vi "ThermoV_ControlSweep_2VO_160717.vi"() -> ()   [LabVIEW 2013]
uses:
  <vilib>/Analysis/baseanly.llb/Mean (DBL).vi
  <vilib>/Analysis/NI_AALBase.lvlib
panel:
  out "time/(60*13) indicator":dbl
  out "VGate Mod10 indicator":dbl
  in  "Operate HVpp\nOutput Timer":bool caption="Reset"
  out "modular 13":dbl
  in  "Number of seconds for \neach HVpp case state":dbl=30.0
  out "Elapsed Time (s)":dbl
  out "DC Value":dbl[](array[numeric]) format="%#.6f"
  in  "How many samples\nto average?":dbl
  in  "Saving Avg?":bool
  in  "Filename":path=path "trial_1.lvm"
  out "Samples Indicator":dbl
  in  "STOP":bool
  in  "Save Waveform":bool
  out "Peak2Peak V":dbl[](array[numeric])
  out "Waveform Chart":dynamicdata(graph)
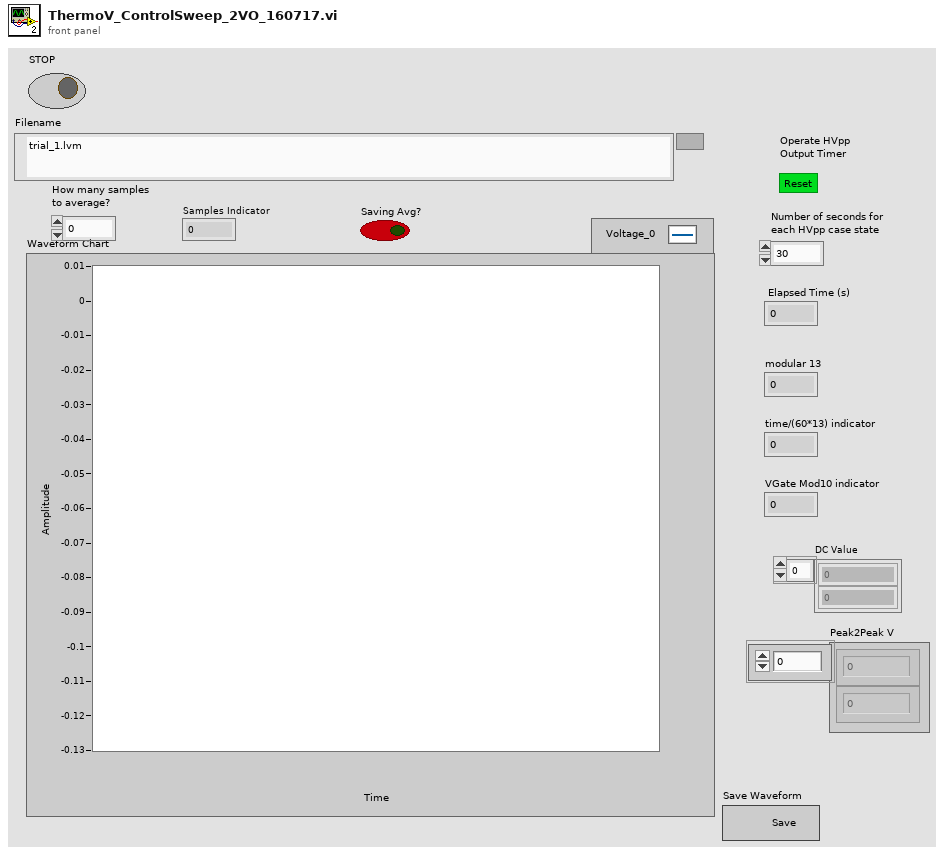
[diagram p1: front panel]
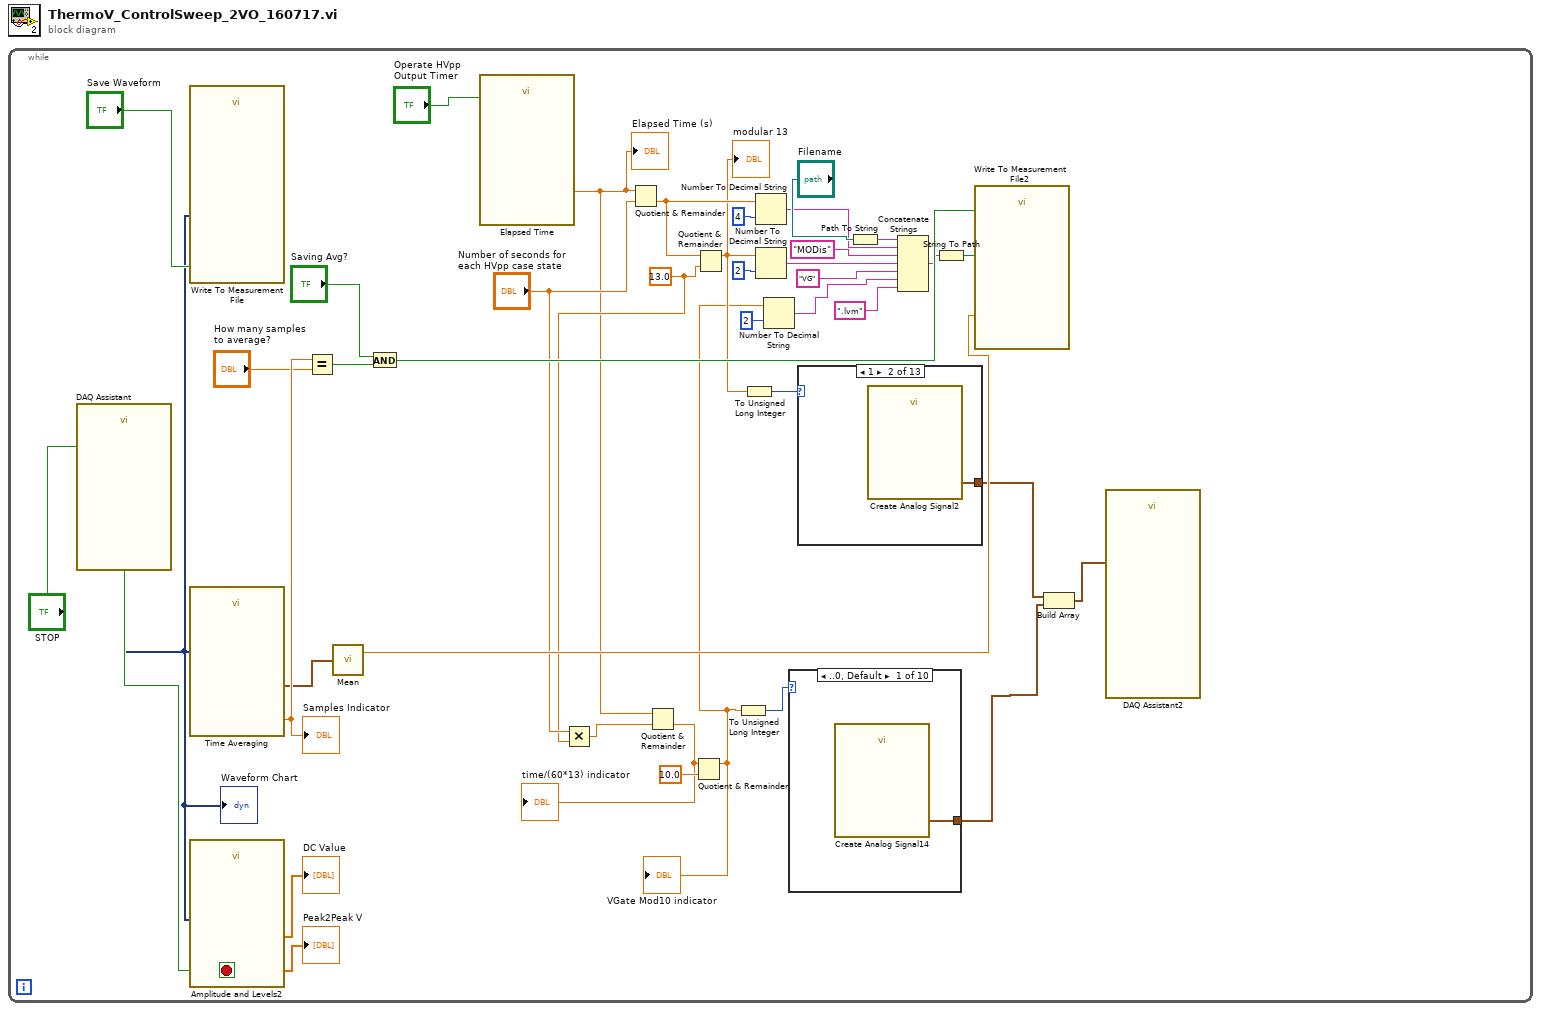
[diagram p0: block diagram]
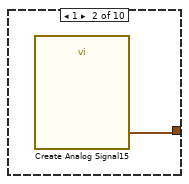
[diagram p2: hidden frame]
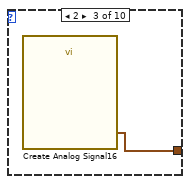
[diagram p3: hidden frame]
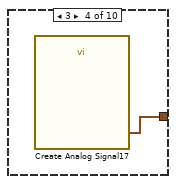
[diagram p4: hidden frame]
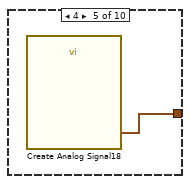
[diagram p5: hidden frame]
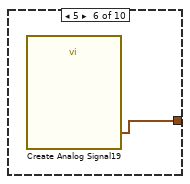
[diagram p6: hidden frame]
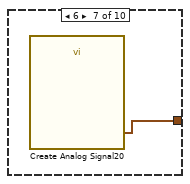
[diagram p7: hidden frame]
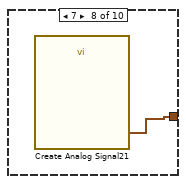
[diagram p8: hidden frame]
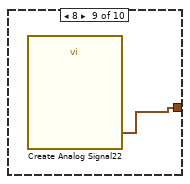
[diagram p9: hidden frame]
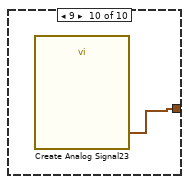
[diagram p10: hidden frame]
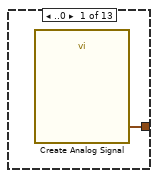
[diagram p11: hidden frame]
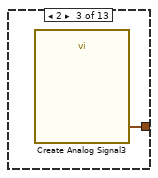
[diagram p12: hidden frame]
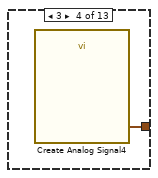
[diagram p13: hidden frame]
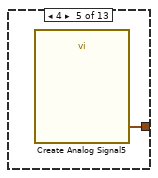
[diagram p14: hidden frame]
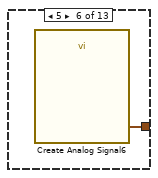
[diagram p15: hidden frame]
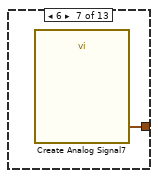
[diagram p16: hidden frame]
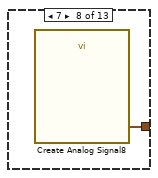
[diagram p17: hidden frame]
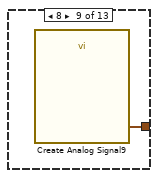
[diagram p18: hidden frame]
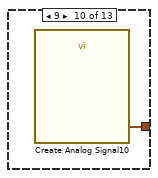
[diagram p19: hidden frame]
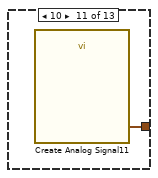
[diagram p20: hidden frame]
diagram:
  n1 = while {
    stop <- w41 stop-if-true
    w13 = 13.0 ("y")
    n2 = call "DAQ Assistant"("stop (F)"="STOP") -> ("data"=w32:dynamicdata, "stopped"=w41:bool)  [unwired: 15 in, 2 out]
    "Waveform Chart" <- w32
    n3 = call "Write To Measurement File"("Signals"=w32, "Enable"="Save Waveform") -> ()  [unwired: 15 in, 3 out]
    n4 = call "Time Averaging"("input signal"=w32) -> ("time avg. signal"=w30:waveform(dbl), "avg. counter"=w37:dbl)  [unwired: 15 in, 2 out]
    "Samples Indicator" <- w37
    n5 = call "Amplitude and Levels2"("input signals"=w32) -> ("dc"=→"DC Value":dbl[], "peak-peak"=→"Peak2Peak V":dbl[])  [unwired: 15 in, 2 out]
    n6 = Equal?(x=w37, y="How many samples\nto average?") -> (x = y?=w35:bool)
    n7 = call-poly <vilib>:"Mean.vi"("X"=w30) -> ("mean"=w29:dbl)  [unwired: 1 out]
    n8 = And(x="Saving Avg?", y=w35) -> (x .and. y?=w34:bool)
    n9 = call "Elapsed Time"("Reset"="Operate HVpp\nOutput Timer") -> ("Elapsed Time (s)"=w12:dbl)  [unwired: 11 in, 7 out]
    "Elapsed Time (s)" <- w12
    n10 = Multiply(x="Number of seconds for \neach HVpp case state", y=w13) -> (x*y=w15:dbl)
    n11 = Quotient & Remainder(x=w12, y="Number of seconds for \neach HVpp case state") -> (floor(x/y)=w22:dbl)  [unwired: 1 out]
    n12 = Quotient & Remainder(x=w12, y=w15) -> (floor(x/y)=w6:dbl)  [unwired: 1 out]
    "time/(60*13) indicator" <- w6
    n13 = Quotient & Remainder(x=w6, y=10.0) -> (x-y*floor(x/y)=w5:dbl)  [unwired: 1 out]
    "VGate Mod10 indicator" <- w5
    n14 = Quotient & Remainder(x=w22, y=w13) -> (x-y*floor(x/y)=w18:dbl)  [unwired: 1 out]
    "modular 13" <- w18
    n15 = To Unsigned Long Integer(number=w5) -> (unsigned 32bit integer=w11:u32)
    n16 = To Unsigned Long Integer(number=w18) -> (unsigned 32bit integer=w28:u32)
    n17 = Number To Decimal String(number=w22, width (-)=i16 4) -> (decimal integer string=w21:string)
    n18 = Number To Decimal String(number=w18, width (-)=i16 2) -> (decimal integer string=w17:string)
    n19 = Number To Decimal String(number=w5, width (-)=i16 2) -> (decimal integer string=w8:string)
    n20 = case shown="..0, Default" w11 {
      tunnel: [w42 w43 w44 w45 w46 w47 w48 w49 w50 w51] -> w3
      frame ..0, Default {
        n21 = call "Create Analog Signal14"() -> ("DC signal"=w42:waveform(dbl))  [unwired: 18 in, 1 out]
      }
      frame 1 {
        n22 = call "Create Analog Signal15"() -> ("DC signal"=w43:waveform(dbl))  [unwired: 18 in, 1 out]
      }
      frame 2 {
        n23 = call "Create Analog Signal16"() -> ("DC signal"=w44:waveform(dbl))  [unwired: 18 in, 1 out]
      }
      frame 3 {
        n24 = call "Create Analog Signal17"() -> ("DC signal"=w45:waveform(dbl))  [unwired: 18 in, 1 out]
      }
      frame 4 {
        n25 = call "Create Analog Signal18"() -> ("DC signal"=w46:waveform(dbl))  [unwired: 18 in, 1 out]
      }
      frame 5 {
        n26 = call "Create Analog Signal19"() -> ("DC signal"=w47:waveform(dbl))  [unwired: 18 in, 1 out]
      }
      frame 6 {
        n27 = call "Create Analog Signal20"() -> ("DC signal"=w48:waveform(dbl))  [unwired: 18 in, 1 out]
      }
      frame 7 {
        n28 = call "Create Analog Signal21"() -> ("DC signal"=w49:waveform(dbl))  [unwired: 18 in, 1 out]
      }
      frame 8 {
        n29 = call "Create Analog Signal22"() -> ("DC signal"=w50:waveform(dbl))  [unwired: 18 in, 1 out]
      }
      frame 9 {
        n30 = call "Create Analog Signal23"() -> ("DC signal"=w51:waveform(dbl))  [unwired: 18 in, 1 out]
      }
    }
    n31 = case shown="1" w28 {
      tunnel: [w52 w53 w54 w55 w56 w57 w58 w59 w60 w61 w62 w63 w64] -> w4
      frame ..0 {
        n32 = call "Create Analog Signal"() -> ("sine wave"=w52:waveform(dbl))  [unwired: 18 in, 1 out]
      }
      frame 1 {
        n33 = call "Create Analog Signal2"() -> ("sine wave"=w53:waveform(dbl))  [unwired: 18 in, 1 out]
      }
      frame 2 {
        n34 = call "Create Analog Signal3"() -> ("sine wave"=w54:waveform(dbl))  [unwired: 18 in, 1 out]
      }
      frame 3 {
        n35 = call "Create Analog Signal4"() -> ("sine wave"=w55:waveform(dbl))  [unwired: 18 in, 1 out]
      }
      frame 4 {
        n36 = call "Create Analog Signal5"() -> ("sine wave"=w56:waveform(dbl))  [unwired: 18 in, 1 out]
      }
      frame 5 {
        n37 = call "Create Analog Signal6"() -> ("sine wave"=w57:waveform(dbl))  [unwired: 18 in, 1 out]
      }
      frame 6 {
        n38 = call "Create Analog Signal7"() -> ("sine wave"=w58:waveform(dbl))  [unwired: 18 in, 1 out]
      }
      frame 7 {
        n39 = call "Create Analog Signal8"() -> ("sine wave"=w59:waveform(dbl))  [unwired: 18 in, 1 out]
      }
      frame 8 {
        n40 = call "Create Analog Signal9"() -> ("sine wave"=w60:waveform(dbl))  [unwired: 18 in, 1 out]
      }
      frame 9 {
        n41 = call "Create Analog Signal10"() -> ("sine wave"=w61:waveform(dbl))  [unwired: 18 in, 1 out]
      }
      frame 10 {
        n42 = call "Create Analog Signal11"() -> ("sine wave"=w62:waveform(dbl))  [unwired: 18 in, 1 out]
      }
      frame 11 {
        n43 = call "Create Analog Signal12"() -> ("sine wave"=w63:waveform(dbl))  [unwired: 18 in, 1 out]
      }
      frame 12.. {
        n44 = call "Create Analog Signal13"() -> ("sine wave"=w64:waveform(dbl))  [unwired: 18 in, 1 out]
      }
    }
    n45 = Path To String(path="Filename") -> (string=w24:string)
    n46 = Concatenate Strings(w24, w21, "MODis" ("string"), w17, "VG" ("string"), w8, ".lvm" ("string")) -> (w25:string)
    n47 = String To Path(string=w25) -> (path=w26:path)
    n48 = call "Write To Measurement File2"("Signals"=w29, "Enable"=w34, "Filename"=w26) -> ()  [unwired: 14 in, 3 out]
    n49 = Build Array(w4, w3) -> (w2:waveform(dbl)[])
    n50 = call "DAQ Assistant2"("data"=w2) -> ()  [unwired: 16 in, 3 out]
  }
